vi "SSC Relay Control Multiple Actions Per-Site.vi"(0 "SSC Relay in":T1[](array[typedef]), 5 "Relay Actions":T3[](array[typedef]) items=["Open Relay"=20, "Close Relay"=21], 7 "Settling Time (s)":dbl format="%#_12p", 9 "Sites":i32[](array[numeric]), 11 "error in":errorcluster) -> (4 "SSC Relay out":T1[](array[typedef]), 8 "Completed Relay Operations":T2[](array[typedef]) {"Desired State" items=["Open Relay"=20, "Close Relay"=21]}, 15 "error out":errorcluster)   [LabVIEW 2019]
doc: "Performs the specified relay action for each Relay associated with the sites that are configured in the SSC Relay session. The function will then wait a specified amount of time if the Settling Time (s) input is wired. \n\nThere must be at exactly one Relay Action per site provided by the Sites input, otherwise the function will return an error."
uses:
  SSC Relay.ctl
  <instrlib>/niSwitch/niSwitch.llb/niSwitch Relay Action.ctl
  SubVIs/TSM Relay Completed Operations.ctl
  SSC Relay Control Core.vi
  Single SSC Relay NI-Switch Control.vi
  Single SSC Relay Fill Additional Error info.vi
  SSC Relay Expand Action Array to All Sessions.vi
  <instrlib>/niSwitch/niSwitch.llb/niSwitch Get Relay Position.vi
  <instrlib>/niSwitch/niSwitch.llb/niSwitch Relay Control.vi
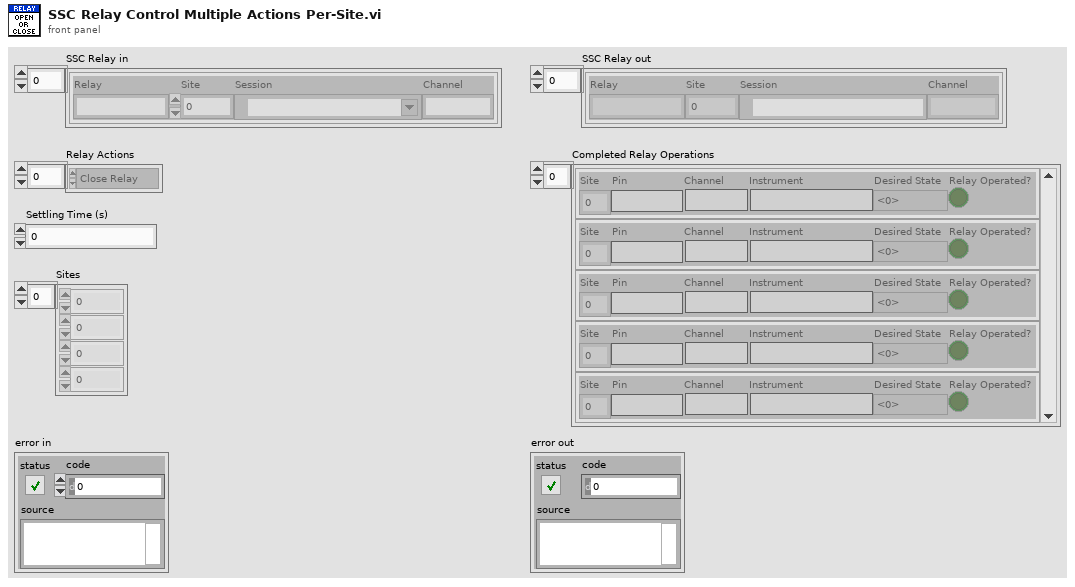
[diagram p1: front panel]
types:
  T1 = typedef "SSC Relay.ctl" = cluster{"Relay":string, "Site":i32, "Session":refnum<k15>, "Channel":string}
  T2 = typedef "TSM Relay Completed Operations.ctl" = cluster{"Site":i32, "Pin":string, "Channel":string, "Instrument":string, "Desired State":T3, "Relay Operated?":bool}
  T3 = typedef "niSwitch Relay Action.ctl" = i32
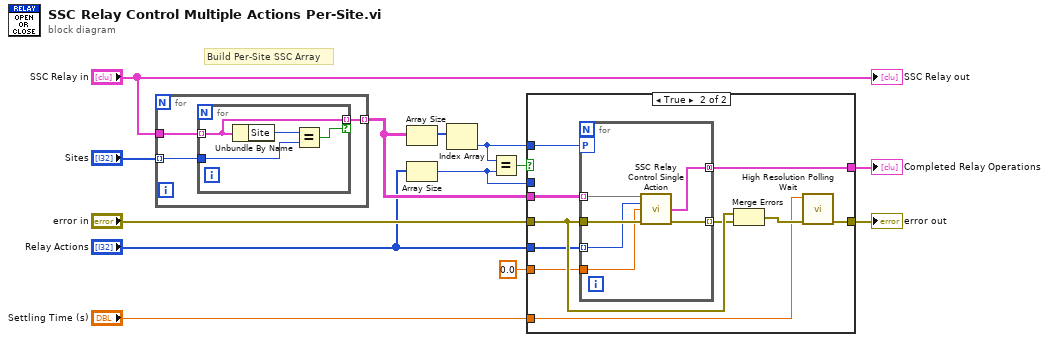
[diagram p0: block diagram]
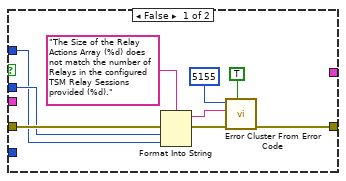
[diagram p2: hidden frame]
diagram:
  # "Build Per-Site SSC Array"
  n1 = for {
    tunnel: "SSC Relay in" -> [w16]
    tunnel: [w15] -> w4 mode=indexing
    tunnel: "Sites" -> [w14] mode=indexing
    n2 = for {
      tunnel: w16 -> [w20] mode=indexing
      tunnel: [w20] -> w15 mode=indexing if=w18
      tunnel: w14 -> [w17]
      n3 = Unbundle By Name(w20) -> ("Site"=w19:i32)
      n4 = Equal?(x=w19, y=w17) -> (x = y?=w18:bool)
    }
  }
  n5 = Array Size(array=w4) -> (size(s)=w13:i32[])
  n6 = Array Size(array="Relay Actions") -> (size(s)=w10:i32)
  n7 = Index Array(array=w13) -> (element=w11:i32)  [unwired: 1 in]
  n8 = Equal?(x=w11, y=w10) -> (x = y?=w12:bool)
  n9 = case shown="True" w12 {
    tunnel: [w26 w38] -> w6
    tunnel: 0.0 ("Settling Time (s)") -> [_ w37]
    tunnel: "error in" -> [w27 w39]
    tunnel: [_ w36] -> w5
    tunnel: "Settling Time (s)" -> [_ w30]
    tunnel: w4 -> [_ w35]
    tunnel: "Relay Actions" -> [_ w34]
    tunnel: w11 -> [w21 w33]
    tunnel: w10 -> [w22 _]
    frame False {
      n10 = Format Into String(format string="The Size of the Relay Actions Array (%d) does not match the number of Relays in the configured TSM Relay Sessions provided (%d)." ("error message (\"\")"), error in=w27, w22, w21) -> (resulting string=w23:string, error out=w25:errorcluster)  [unwired: 1 in]
      n11 = call <vilib>:"Error Cluster From Error Code.vi"("show call chain? (False)"=TRUE, "error in (no error)"=w25, "error message (\"\")"=w23, "error code (0)"=5155) -> ("error out"=w26:errorcluster)  [unwired: 5 in]
    }
    frame True {
      n12 = for {
        tunnel: w37 -> [w40]
        tunnel: w35 -> [w42] mode=indexing
        tunnel: [w41] -> w36 mode=concatenating
        tunnel: w34 -> [w43] mode=indexing
        workers-P: w33 -> [_]
        tunnel: w39 -> [w45]
        tunnel: [w44] -> w31 mode=indexing
        n13 = call "SSC Relay Control Single Action.vi"("SSC Relay in"=w42, "Relay Action"=w43, "Settling Time (s)"=w40, "error in"=w45) -> ("Completed Relay Operations"=w41:T2[], "error out"=w44:errorcluster)  [unwired: 9 in, 1 out]
      }
      n14 = Merge Errors(w39, w31) -> (w32:errorcluster)
      n15 = call <vilib>:"High Resolution Polling Wait.vi"("error in (no error)"=w32, "seconds to wait"=w30) -> ("error out"=w38:errorcluster)  [unwired: 9 in]
    }
  }
  "error out" <- w6
  "Completed Relay Operations" <- w5
  "SSC Relay out" <- "SSC Relay in"
